vi "Write salTypedefPath.vi"(10 "salTypedefPath":path=path "C:/LSSTSW/SAL_LabVIEW_Interface/SALTypedefs/Control 2.ctl", 11 "PolymorphicInstance in":refnum<class "PolymorphicInstance.lvclass">) -> (3 "PolymorphicInstance out":refnum<class "PolymorphicInstance.lvclass">)   [LabVIEW 2012, in "PolymorphicInstance.lvclass"]
uses:
  PolymorphicInstance.lvclass
  PolymorphicInstance.lvclass/PolymorphicInstance.ctl
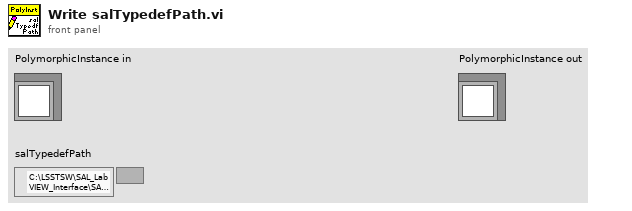
[diagram p1: front panel]
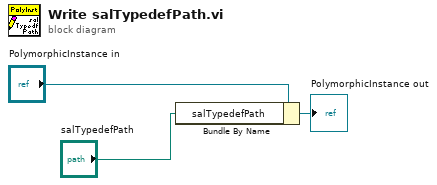
[diagram p0: block diagram]
diagram:
  n1 = Bundle By Name(cluster="PolymorphicInstance in", "salTypedefPath"="salTypedefPath") -> (→"PolymorphicInstance out":refnum<class "PolymorphicInstance.lvclass">)
